vi "Modified Sync Filter Array.vi"(8 "Error In":errorcluster, 9 "order  (3)":i32=3, 10 "side points (6)":i32=6, 11 "Array":dbl[](array[numeric])) -> (0 "Error Out":errorcluster, 3 "Filtered Array":dbl[](array[numeric]))   [LabVIEW 2021, in "Math.lvlib"]
uses:
  Math.lvlib
  <vilib>/Analysis/2dsp.llb/1D Convolution (DBL).vi
  <vilib>/Analysis/NI_AALPro.lvlib
  Error/Error.lvlib
panel:
  # "see the License on the block diagram (Ctrl+E or Window:Show Block Diagram)"
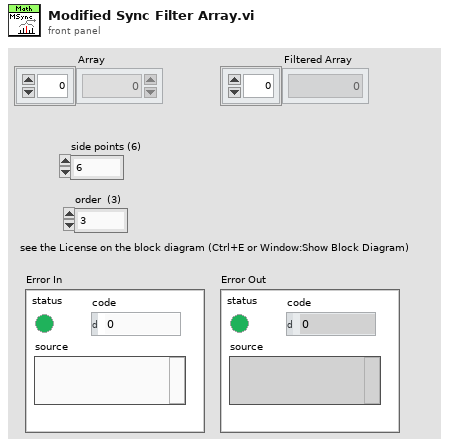
[diagram p1: front panel]
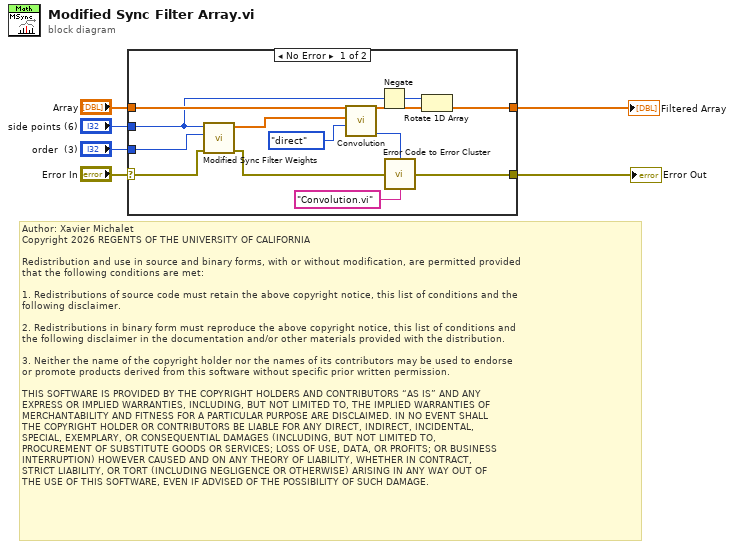
[diagram p0: block diagram]
diagram:
  # "Author: Xavier Michalet\nCopyright 2026 REGENTS OF THE UNIVERSITY OF CALIFORNIA\n\nRedistribution and use in source and binary forms, with or without modification, are permitted provided\nthat the following conditions are met:\n\n1. Redistributions of source code must retain the above copyright notice, this list of conditions and the\nfollowing disclaimer.\n\n2. Redistributions in binary form must reproduce the above copyright notice, this list of conditions and\nthe following disclaimer in the documentation and/or other materials provided with the distribution.\n\n3. Neither the name of the copyright holder nor the names of its contributors may be used to endorse \nor promote products derived from this software without specific prior written permission.\n\nTHIS SOFTWARE IS PROVIDED BY THE COPYRIGHT HOLDERS AND CONTRIBUTORS “AS IS” AND ANY \nEXPRESS OR IMPLIED WARRANTIES, INCLUDING, BUT NOT LIMITED TO, THE IMPLIED WARRANTIES OF\nMERCHANTABILITY AND FITNESS FOR A PARTICULAR PURPOSE ARE DISCLAIMED. IN NO EVENT SHALL\nTHE COPYRIGHT HOLDER OR CONTRIBUTORS BE LIABLE FOR ANY DIRECT, INDIRECT, INCIDENTAL, \nSPECIAL, EXEMPLARY, OR CONSEQUENTIAL DAMAGES (INCLUDING, BUT NOT LIMITED TO, \nPROCUREMENT OF SUBSTITUTE GOODS OR SERVICES; LOSS OF USE, DATA, OR PROFITS; OR BUSINESS\nINTERRUPTION) HOWEVER CAUSED AND ON ANY THEORY OF LIABILITY, WHETHER IN CONTRACT, \nSTRICT LIABILITY, OR TORT (INCLUDING NEGLIGENCE OR OTHERWISE) ARISING IN ANY WAY OUT OF\nTHE USE OF THIS SOFTWARE, EVEN IF ADVISED OF THE POSSIBILITY OF SUCH DAMAGE."
  n1 = case shown="No Error" "Error In" {
    selector: "Error In" -> [w12 w21]
    tunnel: [w17 w21] -> w5
    tunnel: "side points (6)" -> [w8 _]
    tunnel: "order  (3)" -> [w14 _]
    tunnel: "Array" -> [w19 w20]
    tunnel: [w9 w20] -> w1
    frame No Error {
      n2 = call "Modified Sync Filter Weights.vi"("error in (no error)"=w12, "order (n)"=w14, "side points (m)"=w8) -> ("error out"=w11:errorcluster, "weights"=w13:dbl[])  [unwired: 7 in]
      n3 = call-poly <vilib>:"Convolution.vi"("algorithm"=enum32{"direct", "frequency domain"}."direct", "Y"=w13, "X"=w19) -> ("error"=w16:i32, "X * Y"=w18:dbl[])  [unwired: 7 in]
      n4 = Negate(x=w8) -> (-x=w7:i32)
      n5 = call "Error Code to Error Cluster.vi"("Error Code"=w16, "Error Source"="Convolution.vi", "Error In"=w11) -> ("Error Out"=w17:errorcluster)  [unwired: 12 in]
      n6 = Rotate 1D Array(1:w18, 2:w7) -> (0:w9:dbl[])
    }
    frame Error {
    }
  }
  "Error Out" <- w5
  "Filtered Array" <- w1
